vi "Load Layout.vi"(8 "error in (no error)":errorcluster, 11 "TabCtl":refnum<vi>[](array[refnum])) -> (0 "error out":errorcluster)   [LabVIEW 2020, in "MDI ViewManager.lvlib"]
uses:
  MDI ViewManager.lvlib
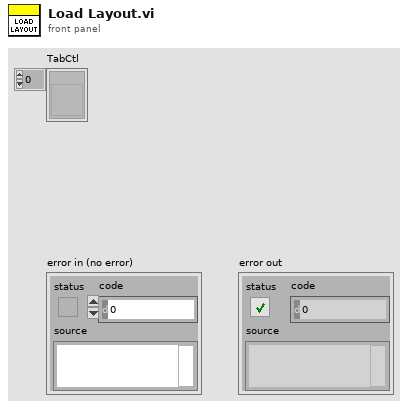
[diagram p1: front panel]
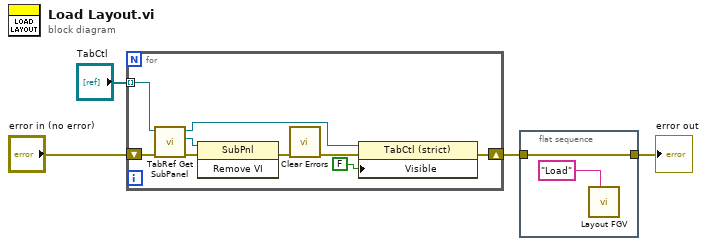
[diagram p0: block diagram]
diagram:
  n1 = for {
    tunnel: "TabCtl" -> [w9] mode=indexing
    shift-right: [w6] -> w1
    shift-left: "error in (no error)" -> [w7]
    n2 = call "TabRef Get SubPanel.vi"("error in (no error)"=w7, "TabControl in"=w9) -> ("error out"=w8:errorcluster, "Sub Panel"=w10:refnum<vi>, "TabControl out"=w5:refnum<vi>)  [unwired: 7 in]
    n3 = invoke class="SubPnl" method="Remove VI"(reference=w10, error in=w8) -> (error out=w12:errorcluster)  [unwired: 1 in, 2 out]
    n4 = call <vilib>:"Clear Errors.vi"("error in (no error)"=w12) -> ("error out"=w11:errorcluster)  [unwired: 5 in, 1 out]
    n5 = property class="TabCtl (strict)"(reference=w5, error in=w11, "Visible"=FALSE) -> (error out=w6:errorcluster)  [unwired: 1 out]
  }
  n6 = flat-sequence {
    tunnel: w1 -> [w15]
    tunnel: [w15] -> w3
    frame #0 {
      n7 = call "Layout FGV.vi"("String"="Load") -> ()  [unwired: 11 in]
    }
  }
  "error out" <- w3
